vi "Get Minimum LabVIEW Version.vi"(8 "error in (no error)":errorcluster, 11 "RSI Module in":refnum<class "RSI Module.lvclass">) -> (0 "error out":errorcluster, 2 "Minimum LabVIEW Version":i32, 3 "RSI Module out":refnum<class "RSI Module.lvclass">)   [LabVIEW 2020, in "Modules.lvlib" / "RSI Module.lvclass"]
uses:
  RSI Module.lvclass
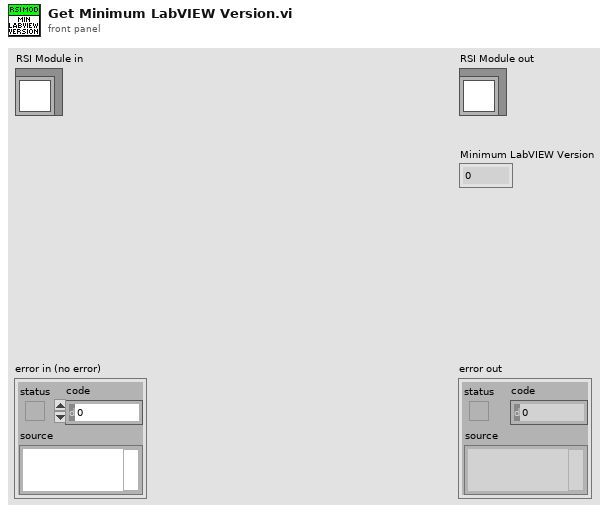
[diagram p1: front panel]
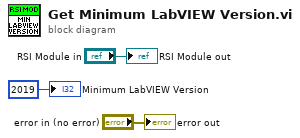
[diagram p0: block diagram]
diagram:
  "error out" <- "error in (no error)"
  "RSI Module out" <- "RSI Module in"
  "Minimum LabVIEW Version" <- 2019 ("Minimum LabVIEW Version")
